vi "Get Min and Max from Range.vi"(8 "error in (no error)":errorcluster, 11 "BinXRange":refnum<k24>) -> (0 "error out":errorcluster, 1 "Maximum":u32, 2 "Minimum":u32)   [LabVIEW 2020]
uses:
  C:/GEECS/Developers Version/builds/Device builds/ThorlabsCsCamera/Thorlabs.TSI.CoreInterfaces.dll
  Thorlabs.TSI.CoreInterfaces.dll
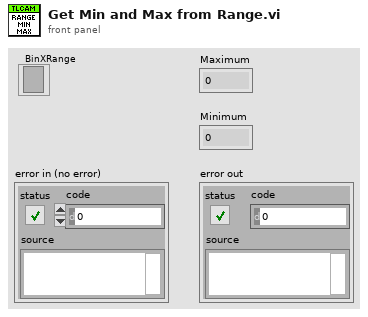
[diagram p1: front panel]
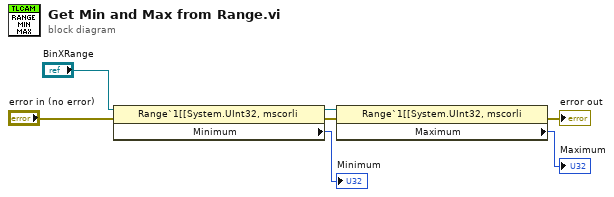
[diagram p0: block diagram]
diagram:
  n1 = property class="Range`1[[System.UInt32, mscorli"(reference="BinXRange", error in="error in (no error)") -> (reference out=w3:refnum<k24>, error out=w4:errorcluster, "Minimum"=→"Minimum":u32)
  n2 = property class="Range`1[[System.UInt32, mscorli"(reference=w3, error in=w4) -> (error out=→"error out":errorcluster, "Maximum"=→"Maximum":u32)  [unwired: 1 out]
